vi "Work.vi"(9 "In":cluster{"t0":dbl, "dt":dbl, "y":cdb[]}, 11 "Action":T1) -> (1 "Out":cluster{"t0":dbl, "dt":dbl, "y":dbl[]})   [LabVIEW 2020, in "AAL-FFT CDB.lvlib"]
uses:
  AAL-FFT CDB.lvlib
  Block/FlexBlocks/Worker Action.ctl
  <vilib>/Analysis/2dsp.llb/Complex FFT.vi
  <vilib>/Analysis/NI_AALPro.lvlib
  Block/FlexBlocks/FlexBlocks.lvlib
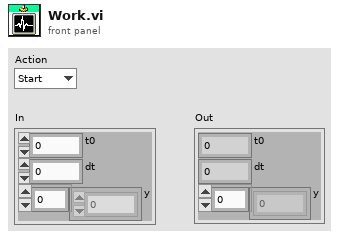
[diagram p1: front panel]
types:
  T1 = typedef "FlexBlocks.lvlib/Worker Action.ctl" = enum16{"Start", "Work", "Stop"}
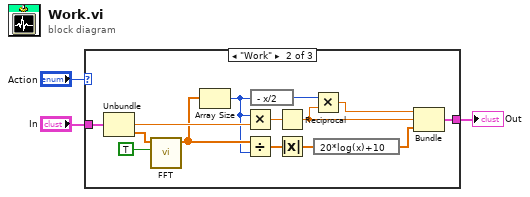
[diagram p0: block diagram]
diagram:
  n1 = case shown="\"Work\"" "Action" {
    tunnel: "In" -> [_ w17 _]
    tunnel: [_ w4 _] -> w1
    frame "Start" {
    }
    frame "Work" {
      n2 = Unbundle(w17) -> ("dt"=w14:dbl, "y"=w15:cdb[])  [unwired: 1 out]
      n3 = call-poly <vilib>:"FFT.vi"("shift?"=TRUE, "X"=w15) -> ("FFT {X}"=w9:cdb[])  [unwired: 8 in, 1 out]
      n4 = Array Size(array=w9) -> (size(s)=w8:i32)
      n5 = Multiply(x=w8, y=w14) -> (x*y=w13:dbl)
      n6 = Divide(x=w9, y=w8) -> (x/y=w7:cdb[])
      n7 = expression code="- x/2"(w8) -> (w12:i32)
      n8 = Reciprocal(x=w13) -> (1/x=w10:dbl)
      n9 = Absolute Value(x=w7) -> (abs(x)=w6:dbl[])
      n10 = Multiply(x=w12, y=w10) -> (x*y=w11:dbl)
      n11 = expression code="20*log(x)+10"(w6) -> (w5:dbl[])
      n12 = Bundle(w11, w10, w5) -> (w4:cluster{dbl, dbl, dbl[]})  [unwired: 1 in]
    }
    frame "Stop" {
    }
  }
  "Out" <- w1
